vi "Run Tests.vi"() -> ()   [LabVIEW 2014, in "SQLite3LV Tests.lvlib"]
uses:
  SQLite3LV Tests.lvlib
panel:
  out "progress":u8(slide) scale=0.0..100.0
  in  "Multicolumn Listbox":i32(listbox)
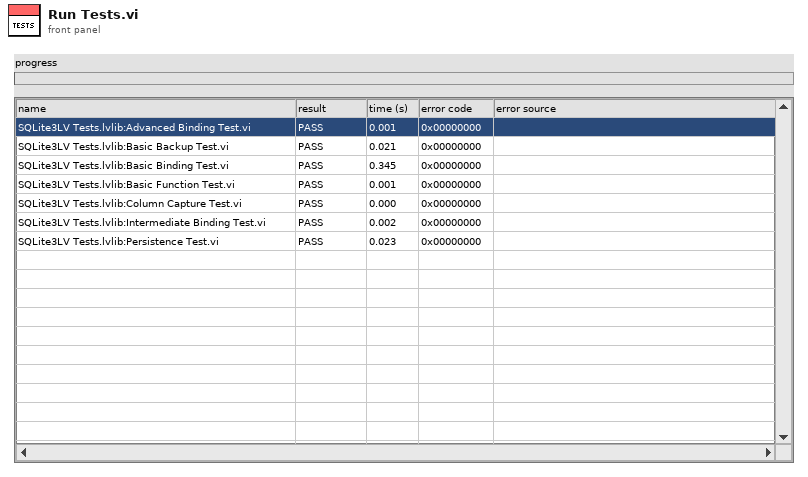
[diagram p1: front panel]
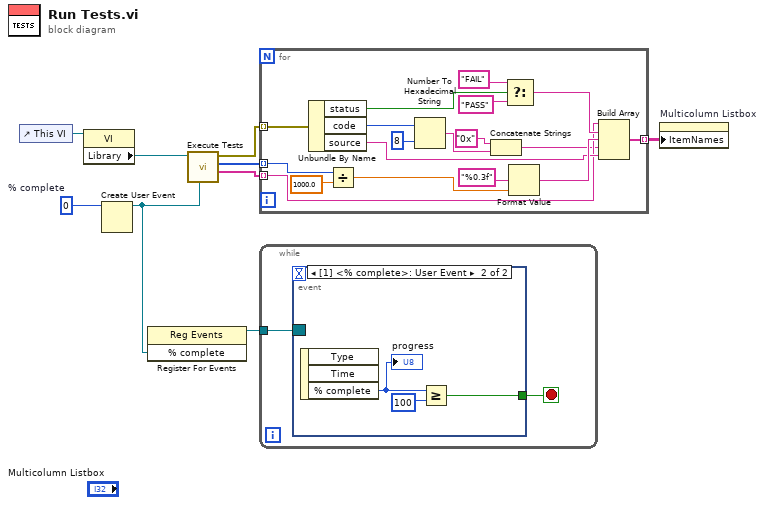
[diagram p0: block diagram]
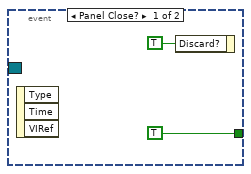
[diagram p2: hidden frame]
diagram:
  w2 = 0  # % complete
  n1 = control-ref of="This VI"() -> (w9:refnum<vi>)
  n2 = property class="VI"(reference=w9) -> ("Library"=w8:refnum<vi>)  [unwired: 1 in, 2 out]
  n3 = Create User Event(user event datatype=w2) -> (user event=w1:refnum<user-event>)  [unwired: 1 in, 1 out]
  n4 = register-events(w1) -> (reference out=w3:refnum<event-registration>)  [unwired: 2 in, 1 out]
  n5 = call "Execute Tests.vi"("% complete"=w1, "Library in"=w8) -> ("Tests"=w5:string[], "execution times (ms)"=w6:u32[], "results"=w7:errorcluster[])  [unwired: 7 in]
  n6 = for {
    tunnel: w7 -> [w27] mode=indexing
    tunnel: w6 -> [w21] mode=indexing
    tunnel: [w15] -> w4 mode=indexing
    tunnel: w5 -> [w14] mode=indexing
    n7 = Unbundle By Name(w27) -> ("status"=w26:bool, "code"=w18:i32, "source"=w16:string)
    n8 = Divide(x=w21, y=1000.0) -> (x/y=w13:dbl)
    n9 = Number To Hexadecimal String(1:i16 8 ("width (-)"), 2:w18) -> (0:w17:string)
    n10 = Concatenate Strings("0x" ("string"), w17) -> (w12:string)
    n11 = Select(t="FAIL", s=w26, f="PASS") -> (s? t:f=w23:string)
    n12 = Format Value(format string="%0.3f", value (0)=w13) -> (output string=w19:string)  [unwired: 1 in]
    n13 = Build Array(w14, w23, w19, w12, w16) -> (w15:string[])
  }
  n14 = while {
    tunnel: w3 -> [w29]
    stop <- w28 stop-if-true
    n15 = event shown="[1] <% complete>: User Event" {
      selector: w29 -> [_ _]
      dyn-events: _ -> [_ _]
      timeout: _ -> [_ _]
      tunnel: [TRUE ("Discard?") w32] -> w28
      event Panel Close? {
        n16 = event-data() -> ()  [unwired: 1 in, 3 out]
        n17 = event-data("Discard?"=TRUE) -> ()  [unwired: 1 in, 1 out]
      }
      event User Event {
        n18 = event-data() -> ("% complete"=w34:i32)  [unwired: 1 in, 2 out]
        "progress" <- w34
        n19 = Greater Or Equal?(x=w34, y=100) -> (x >= y?=w32:bool)
      }
    }
  }
  n20 = property on="Multicolumn Listbox" class="MCListbox (strict)"("ItemNames"=w4) -> ()  [unwired: 2 in, 2 out]
